vi "Read FunctionalitiesEvnts.vi"(8 "error in (no error)":errorcluster, 11 "ElectrometerController in":refnum<class "ElectrometerController.lvclass">) -> (0 "error out":errorcluster, 2 "FunctionalitiesEvnts":T1, 3 "ElectrometerController out":refnum<class "ElectrometerController.lvclass">)   [LabVIEW 2016, in "ElectrometerController.lvclass"]
uses:
  ElectrometerController.lvclass
  controls/functionalitiesEvnts.ctl
  Electrometer/Modes.ctl
  ElectrometerController.lvclass/ElectrometerController.ctl
  Electrometer/Electrometer.lvclass
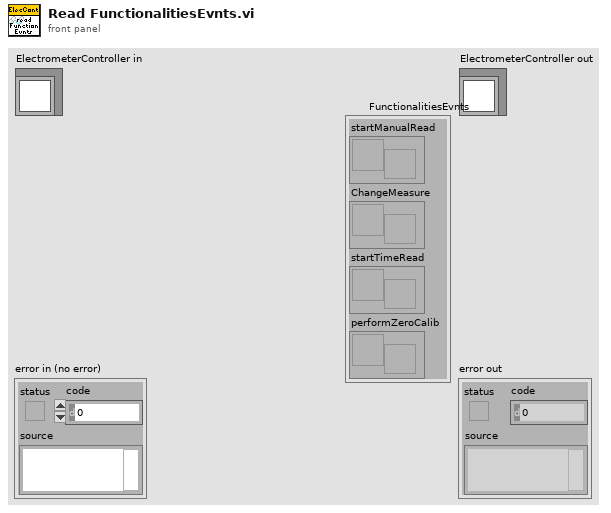
[diagram p1: front panel]
types:
  T1 = typedef "ElectrometerController.lvclass/functionalitiesEvnts.ctl" = cluster{"startManualRead":refnum<user-event>, "ChangeMeasure":refnum<user-event>, "startTimeRead":refnum<user-event>, "performZeroCalib":refnum<user-event>}
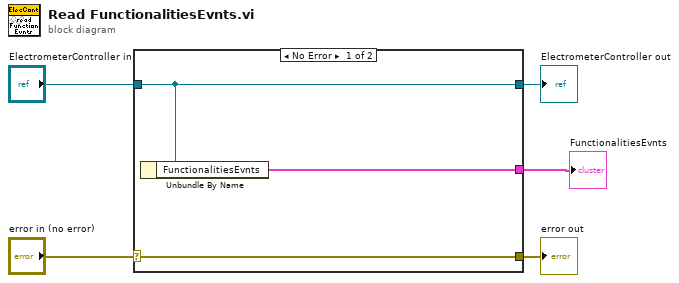
[diagram p0: block diagram]
diagram:
  n1 = case shown="No Error" "error in (no error)" {
    selector: "error in (no error)" -> [w8 w9]
    tunnel: [w8 w9] -> w4
    tunnel: [w7 w10] -> w2
    tunnel: "ElectrometerController in" -> [w7 w10]
    tunnel: [w6 _] -> w1
    frame No Error {
      n2 = Unbundle By Name(w7) -> ("FunctionalitiesEvnts"=w6:T1)
    }
    frame Error {
    }
  }
  "error out" <- w4
  "ElectrometerController out" <- w2
  "FunctionalitiesEvnts" <- w1
